vi "UTIL Probe.vi"(8 "error in (no error)":errorcluster, 11 "niDTS Comm EXE in":refnum<class "niDTS Comm EXE.lvclass">) -> (0 "error out":errorcluster, 3 "niDTS Comm EXE out":refnum<class "niDTS Comm EXE.lvclass">)   [LabVIEW 2015, in "niDTS CommLib.lvlib" / "niDTS Comm EXE.lvclass"]
uses:
  niDTS Comm EXE.lvclass
  Includes/niDTS Comm INC EXE Port Parameters.ctl
  niDTS Comm EXE.lvclass/niDTS Comm EXE.ctl
  niDTS CommLib.lvlib
panel:
  out "Port Parameters":T1={"Timeout (s)"=4096.0}
  out "EXE Path":path
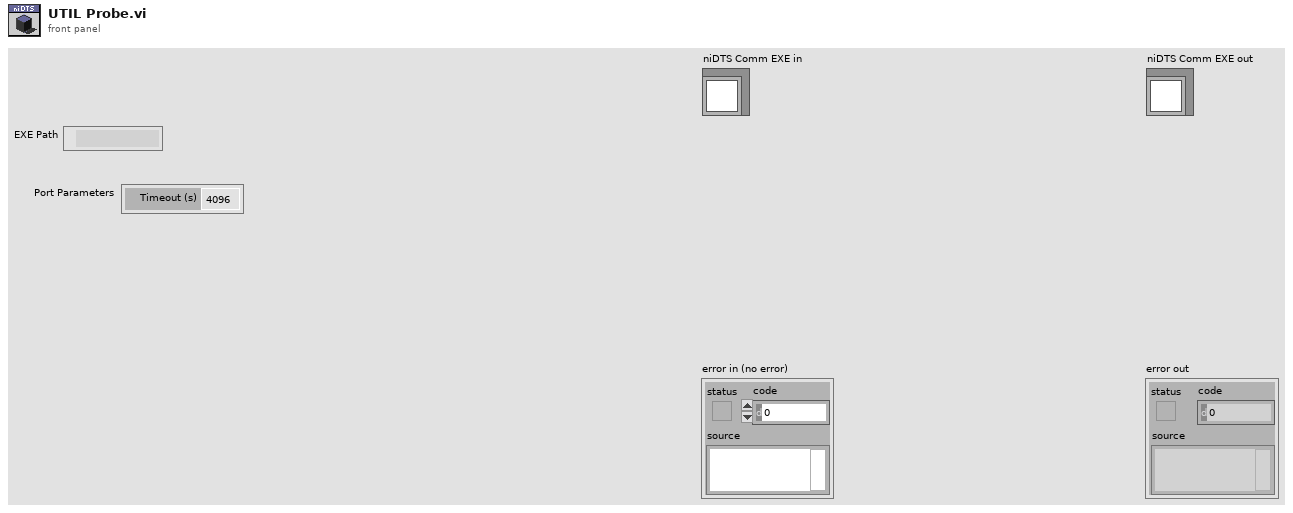
[diagram p1: front panel]
types:
  T1 = typedef "niDTS CommLib.lvlib/niDTS Comm INC EXE Port Parameters.ctl" = cluster{"Timeout (s)":dbl}
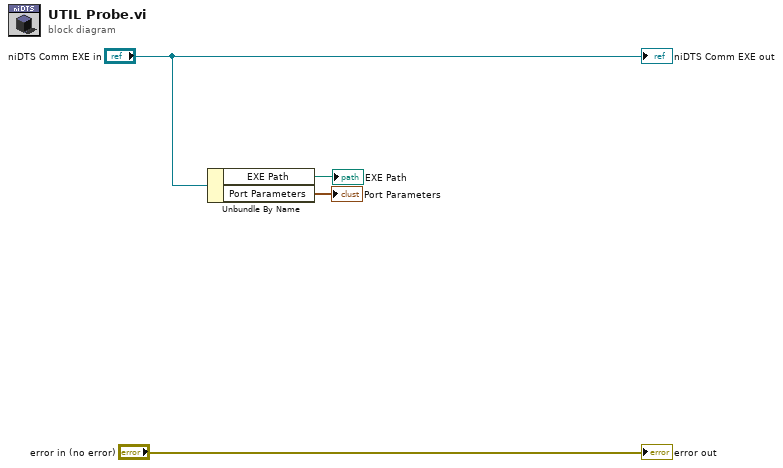
[diagram p0: block diagram]
diagram:
  n1 = Unbundle By Name("niDTS Comm EXE in") -> ("EXE Path"=→"EXE Path":path, "Port Parameters"=→"Port Parameters":T1)
  "error out" <- "error in (no error)"
  "niDTS Comm EXE out" <- "niDTS Comm EXE in"
